vi "Read Humidity DBL.vi"(8 "error in":errorcluster, 10 "Source":string, 11 "IRead Absolute Humidity in":refnum<class "Virtual NEO480.lvclass">) -> (0 "error out":errorcluster, 1 "Time Stamp":timestamp format="%<%x %.3X>T", 2 "Absolute Humidity":dbl format="%.1f g/m³", 3 "IRead Absolute Humidity out":refnum<class "Virtual NEO480.lvclass">)   [LabVIEW 2024, in "Virtual NEO480.lvclass"]
uses:
  Virtual NEO480.lvclass
  D:/git/HAL/Source/Action Point/Action Point.lvclass
  Source/Action Point/Action Point.lvclass/Action Point.ctl
  Virtual NEO480.lvclass/Virtual NEO480.ctl
  Source/Interfaces/ILog Data/ILog Data.lvclass
  Source/DBC Communicator/DBC Communicator.lvclass
  Source/Action Point/Action Point.lvclass
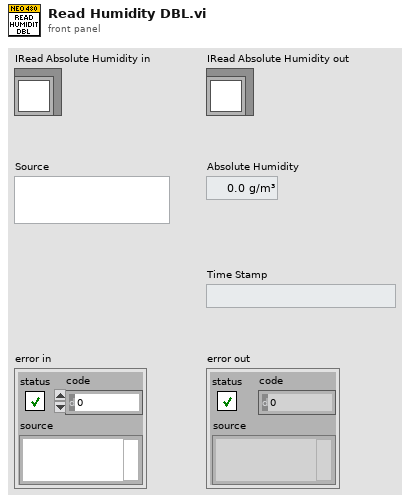
[diagram p1: front panel]
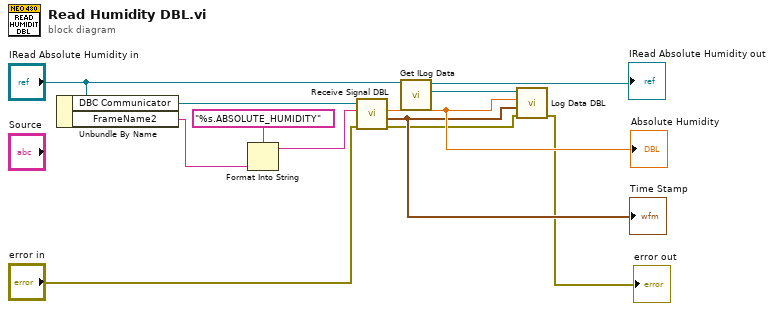
[diagram p0: block diagram]
diagram:
  n1 = Unbundle By Name("IRead Absolute Humidity in") -> ("DBC Communicator"=w10:refnum<class "DBC Communicator.lvclass">, "FrameName2"=w11:string)
  n2 = Format Into String(format string="%s.ABSOLUTE_HUMIDITY", w11) -> (resulting string=w9:string)  [unwired: 2 in, 1 out]
  n3 = call "Receive Signal DBL.vi"("error in"="error in", "Signal Name"=w9, "DBC Communication in"=w10) -> ("error out"=w2:errorcluster, "Time Stamp"=w3:timestamp, "Value"=w4:dbl)  [unwired: 5 in, 1 out]
  "Absolute Humidity" <- w4
  "Time Stamp" <- w3
  n4 = call "Get ILog Data.vi"("Action Point in"="IRead Absolute Humidity in") -> ("ILog Data"=w7:refnum<class "ILog Data.lvclass">, "Action Point out"=→"IRead Absolute Humidity out":refnum<class "Virtual NEO480.lvclass">)  [unwired: 9 in]
  n5 = call-dynamic "Log Data DBL.vi"("error in"=w2, "Time Stamp"=w3, "Data"=w4, "IDataLogger in"=w7) -> ("error out"=→"error out":errorcluster)  [unwired: 6 in, 1 out]
